vi "tearDown.vi"(8 "error in":errorcluster, 11 "logging loopback":refnum<class "Logging Loopback.lvclass">) -> (0 "error out":errorcluster, 3 "logging loopback out":refnum<class "Logging Loopback.lvclass">)   [LabVIEW 2020, in "Logging Loopback.lvclass"]
doc: "tearDown runs after the test method has completed. Use this method to clean up any operations or references that were opened by setUp or the test method. Unit tests should be independent of other unit tests so this VI should ensure that the next test can run in a 'clean' test environment."
uses:
  Logging Loopback.lvclass
  Logging Loopback.lvclass/Logging Loopback.ctl
  <vilib>/WebDAVClient/NI_WebDAV.lvlib
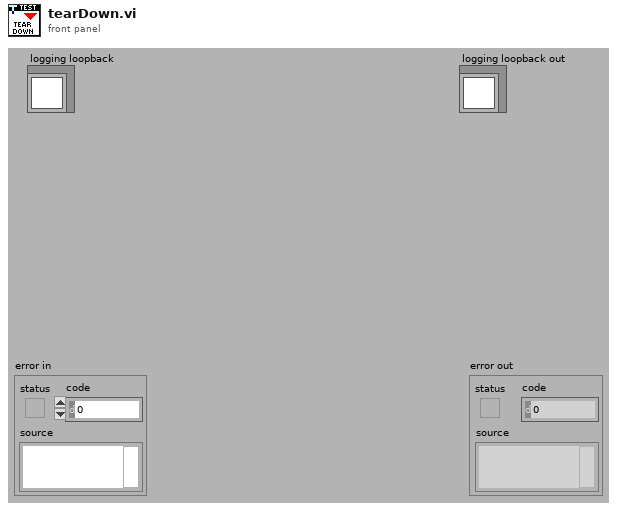
[diagram p1: front panel]
types:
  T1 = typedef "NI_WebDAV.lvlib/SessionHandle.ctl" = refnum<k1>
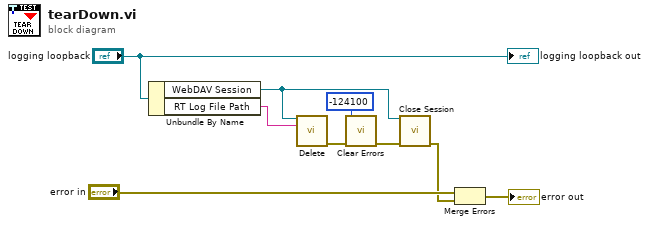
[diagram p0: block diagram]
diagram:
  n1 = Unbundle By Name("logging loopback") -> ("WebDAV Session"=w2:T1, "RT Log File Path"=w4:string)
  n2 = call <vilib>:"Delete.vi"("session handle"=w2, "relative uri"=w4) -> ("error out"=w6:errorcluster)  [unwired: 12 in, 1 out]
  n3 = call <vilib>:"Clear Errors.vi"("error in (no error)"=w6, "specific error code to clear (0: all)"=-124100) -> ("error out"=w3:errorcluster)  [unwired: 4 in, 1 out]
  n4 = call <vilib>:"Close Session.vi"("session handle"=w2, "error in (no error)"=w3) -> ("error out"=w1:errorcluster)  [unwired: 13 in]
  n5 = Merge Errors("error in", w1) -> (→"error out":errorcluster)
  "logging loopback out" <- "logging loopback"
